vi "MyReadTemp.vi"(8 "error in (no error)":errorcluster, 10 "Temperature Channel":i32, 11 "VISA resource name in":refnum<visa-resource-name>="TCPIP0::192.168.0.107::33576::SOCKET") -> (0 "error out":errorcluster, 2 "Temperature":dbl, 3 "VISA resource name out":refnum<visa-resource-name>)   [LabVIEW 2025, in "MyTriton.lvlib"]
uses:
  MyTriton.lvlib
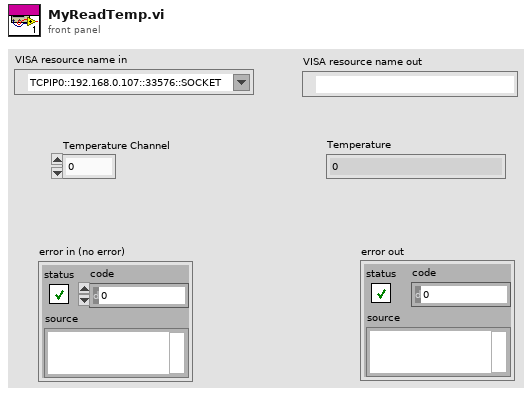
[diagram p1: front panel]
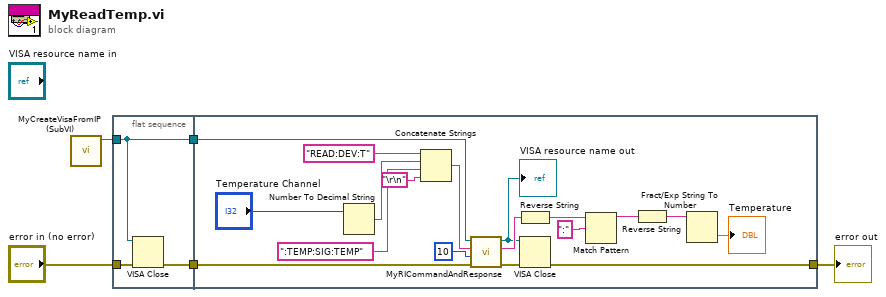
[diagram p0: block diagram]
diagram:
  n1 = call "MyCreateVisaFromIP (SubVI).vi"() -> ("VISA Refnum out"=w1:refnum<visa-resource-name>)  [unwired: 11 in]
  n2 = flat-sequence {
    tunnel: w1 -> [w8]
    tunnel: [w8] -> w3
    tunnel: [w7] -> w2
    tunnel: "error in (no error)" -> [w6]
    tunnel: w3 -> [w13]
    tunnel: w2 -> [w12]
    tunnel: [w9] -> w4
    frame #0 {
      n3 = VISA Close(VISA resource name=w8, error in (no error)=w6) -> (error out=w7:errorcluster)
    }
    frame #1 {
      n4 = Number To Decimal String(number="Temperature Channel") -> (decimal integer string=w24:string)  [unwired: 1 in]
      n5 = Concatenate Strings("READ:DEV:T", w24, ":TEMP:SIG:TEMP", "\r\n") -> (w16:string)
      n6 = call "MyRICommandAndResponse.vi"("error in (no error)"=w12, "Min byte count"=u32 10, "Command"=w16, "VISA resource name in"=w13) -> ("error out"=w10:errorcluster, "Response"=w14:string, "VISA resource name out"=w11:refnum<visa-resource-name>)  [unwired: 5 in]
      "VISA resource name out" <- w11
      n7 = Reverse String(1:w14) -> (0:w21:string)
      n8 = VISA Close(VISA resource name=w11, error in (no error)=w10) -> (error out=w9:errorcluster)
      n9 = Match Pattern(string=w21, regular expression=":") -> (before substring=w19:string)  [unwired: 1 in, 3 out]
      n10 = Reverse String(1:w19) -> (0:w18:string)
      n11 = Fract/Exp String To Number(string=w18) -> (number=→"Temperature":dbl)  [unwired: 3 in, 1 out]
    }
  }
  "error out" <- w4
